vi "fix dll.vi"() -> ()   [LabVIEW 2023]
panel:
  out "Class ID":u32[](array[numeric])
  out "Array":string[](array[string])
  out "Numeric":i32
  in  "vi path 2":path
  out "error out":errorcluster
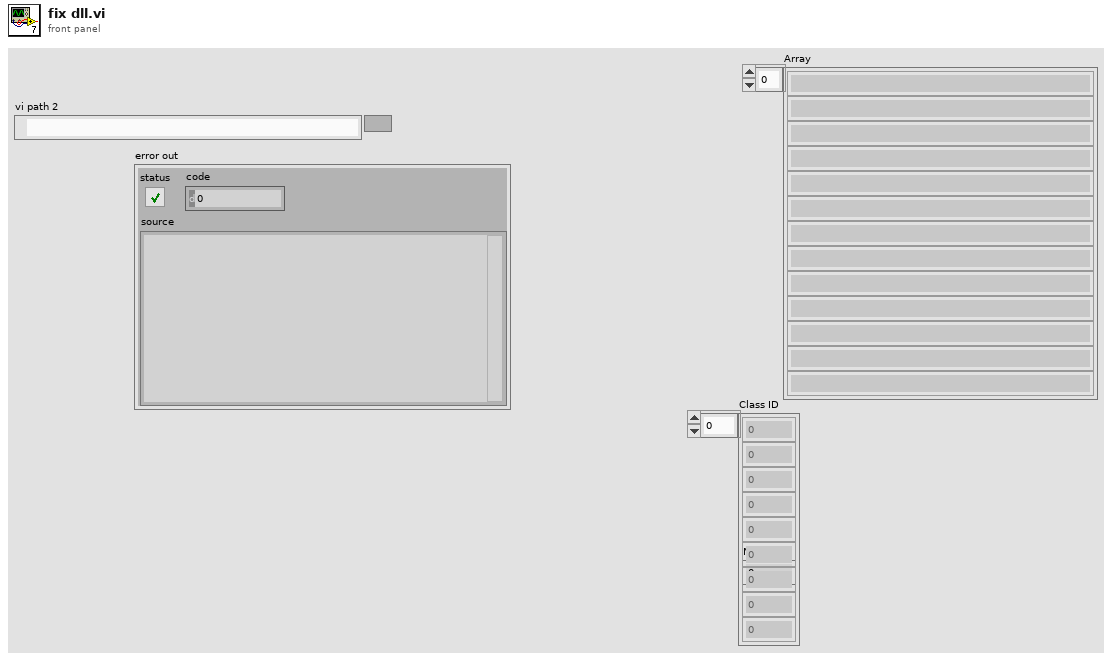
[diagram p1: front panel]
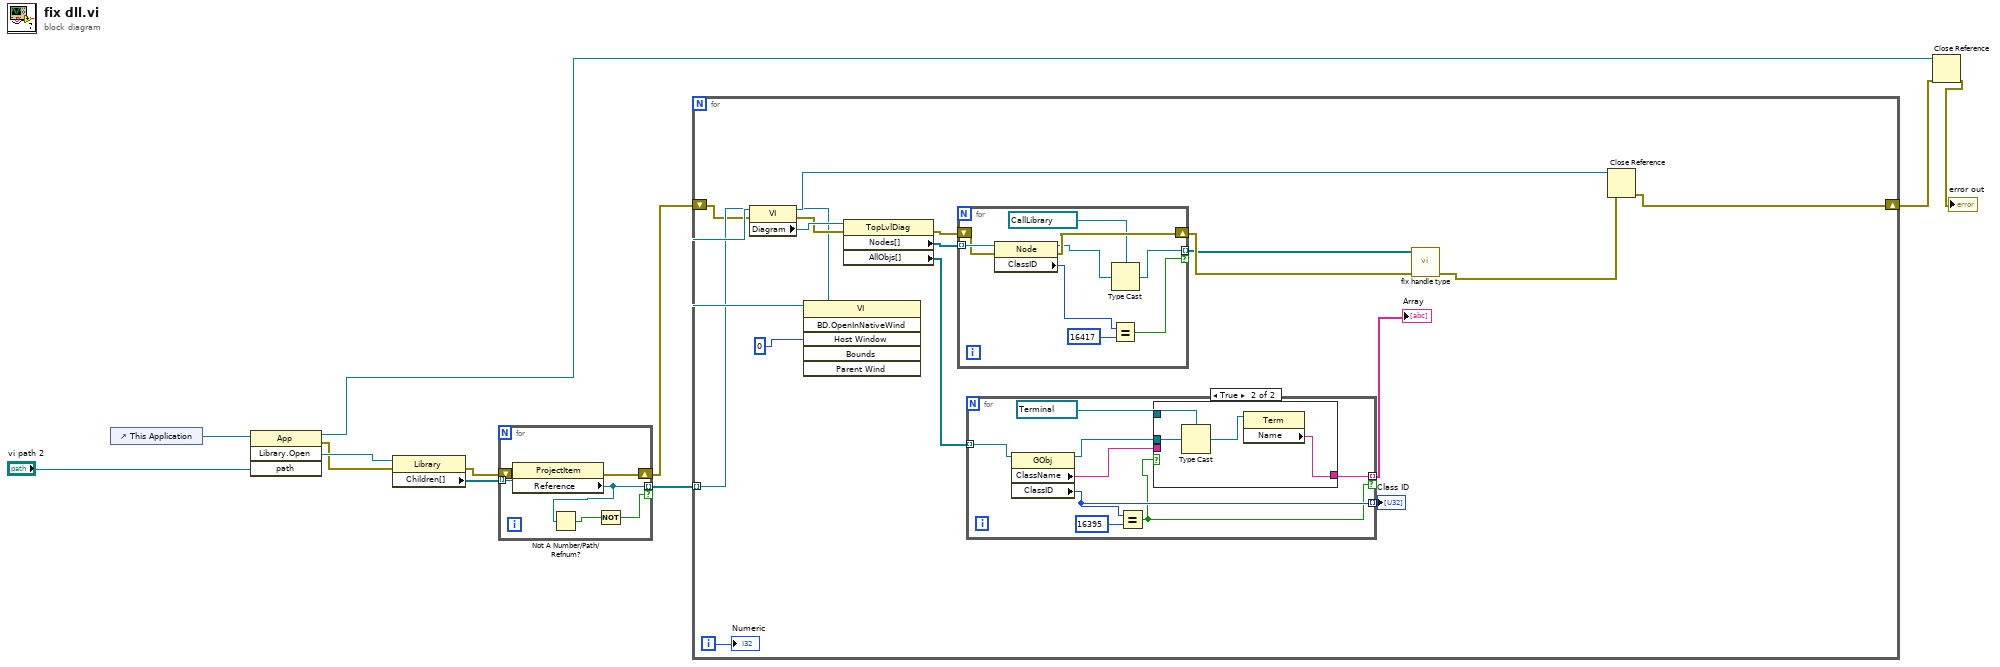
[diagram p0: block diagram]
diagram:
  n1 = control-ref of="This Application"() -> (w11:refnum<vi>)
  n2 = invoke class="App" method="Library.Open"(reference=w11, "path"="vi path 2") -> (reference out=w9:refnum<vi>, error out=w6:errorcluster, "Open Library"=w8:refnum<vi>)  [unwired: 2 in, 1 out]
  n3 = property class="Library"(reference=w8, error in=w6) -> (error out=w4:errorcluster, "Children[]"=w7:refnum<vi>[])  [unwired: 1 out]
  n4 = for {
    tunnel: w7 -> [w17] mode=indexing
    tunnel: [w16] -> w5 mode=indexing if=w14
    shift-right: [w12] -> w3
    shift-left: w4 -> [w13]
    n5 = property class="ProjectItem"(reference=w17, error in=w13) -> (error out=w12:errorcluster, "Reference"=w16:refnum<vi>)  [unwired: 1 out]
    n6 = Not A Number/Path/Refnum?(number/path/refnum=w16) -> (NaN/Path/Refnum?=w15:bool)
    n7 = Not(x=w15) -> (.not. x?=w14:bool)
  }
  n8 = for {
    tunnel: w5 -> [w25] mode=indexing
    shift-right: [w23] -> w2
    shift-left: w3 -> [w22]
    i -> [w21]
    n9 = invoke class="VI" method="BD.OpenInNativeWind"(reference=w25, "Host Window"=u64 0) -> (reference out=w27:refnum<vi>)  [unwired: 4 in, 5 out]
    n10 = property class="VI"(reference=w27, error in=w22) -> (reference out=w32:refnum<vi>, error out=w31:errorcluster, "Diagram"=w34:refnum<vi>)
    n11 = property class="TopLvlDiag"(reference=w34, error in=w31) -> (error out=w30:errorcluster, "Nodes[]"=w33:refnum<vi>[], "AllObjs[]"=w20:refnum<vi>[])  [unwired: 1 out]
    n12 = for {
      tunnel: w33 -> [w55] mode=indexing
      tunnel: [w47] -> w28 mode=indexing if=w50
      shift-right: [w53] -> w29
      shift-left: w30 -> [w54]
      n13 = property class="Node"(reference=w55, error in=w54) -> (reference out=w49:refnum<vi>, error out=w53:errorcluster, "ClassID"=w52:u32)
      n14 = Type Cast(type=refnum<vi> refnum ("reference out"), x=w49) -> (*(type *) &x=w47:refnum<vi>)
      n15 = Equal?(x=w52, y=u32 16417) -> (x = y?=w50:bool)
    }
    n16 = for {
      tunnel: w20 -> [w42] mode=indexing
      tunnel: [w37] -> w19 mode=indexing if=w36
      tunnel: [w40] -> w18 mode=indexing
      n17 = property class="GObj"(reference=w42) -> (reference out=w39:refnum<vi>, "ClassName"=w35:string, "ClassID"=w40:u32)  [unwired: 1 in, 1 out]
      n18 = Equal?(x=w40, y=u32 16395) -> (x = y?=w36:bool)
      n19 = case shown="True" w36 {
        tunnel: w39 -> [_ w46]
        tunnel: refnum<vi> refnum ("reference out") -> [_ w45]
        tunnel: [_ w43] -> w37
        tunnel: w35 -> [_ _]
        frame False {
        }
        frame True {
          n20 = Type Cast(type=w45, x=w46) -> (*(type *) &x=w44:refnum<vi>)
          n21 = property class="Term"(reference=w44) -> ("Name"=w43:string)  [unwired: 1 in, 2 out]
        }
      }
    }
    "Array" <- w19
    "Class ID" <- w18
    n22 = call "fix handle type.vi"("error in (no error)"=w29, "CLF Nodes"=w28) -> ("error out"=w24:errorcluster)  [unwired: 8 in, 1 out]
    n23 = Close Reference(reference=w32, error in (no error)=w24) -> (error out=w23:errorcluster)
    "Numeric" <- w21
  }
  n24 = Close Reference(reference=w9, error in (no error)=w2) -> (error out=→"error out":errorcluster)
